vi "Brandon Connection Test.vi"() -> ()   [LabVIEW 2013]
uses:
  <vilib>/Rock Robotics/SystemInterfaces/DIO/FPGA_DIOChannel.ctl
  <vilib>/Rock Robotics/WPI/SPI/WPI_SPIFrameMode.ctl
  <vilib>/Rock Robotics/WPI/SPI/WPI_SPIBits Per Word.ctl
panel:
  out "Binary":bool[](array[boolean])
  out "Received Data":u32
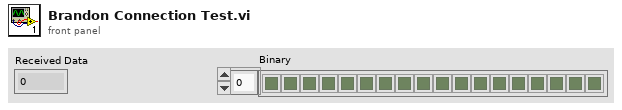
[diagram p1: front panel]
types:
  T1 = typedef "WPI_SPIBits Per Word.ctl" = u8
  T2 = typedef "FPGA_DIOChannel.ctl" = enum8{"DIO 1", "DIO 2", "DIO 3", "DIO 4", "DIO 5", "DIO 6", "DIO 7", "DIO 8", "DIO 9", "DIO 10", "DIO 11", "DIO 12", "DIO 13", "DIO 14", "Invalid"}
  T3 = typedef "WPI_SPIFrameMode.ctl" = enum16{"Chip Select", "Pre-Latch Pulse", "Post-Latch Pulse", "Pre- and Post-Latch Pulse"}
  T4 = typedef "WPI_DigitalOutputDevRef.ctl" = cluster{"Digital Module":T5, "DIO Channel":T2, "DevStatus":errorcluster}
  T5 = typedef "FPGA_TypedefDigitalModule.ctl" = enum16{"Digital Module 1", "Digital Module 2"}
  T6 = typedef "WPI_DigitalInputDevRef.ctl" = cluster{"DevStatus":errorcluster, "DIO Channel":T2, "Digital Module":T5}
  T7 = typedef "WPI_SPIDevRef.ctl" = cluster{"DevStatus":errorcluster}
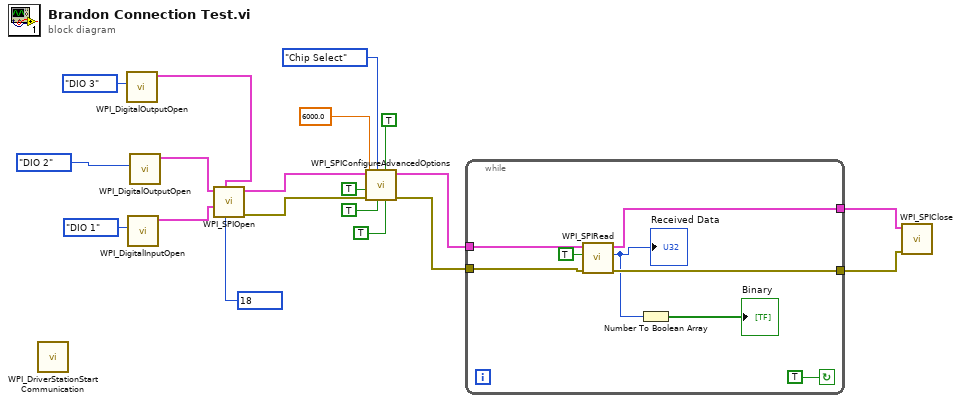
[diagram p0: block diagram]
diagram:
  w1 = T1 18 items=["8-Bit"=8, "16-Bit"=16, "32-Bit"=32] ("Bits Per Word")
  n1 = call <vilib>:"WPI_DriverStationStart Communication.vi"() -> ()  [unwired: 12 in]
  n2 = call <vilib>:"WPI_DigitalOutputOpen.vi"("DIO Channel"=FPGA_DIOChannel."DIO 3") -> ("DigitalOutputDevRef"=w14:T4)  [unwired: 9 in, 1 out]
  n3 = call <vilib>:"WPI_DigitalInputOpen.vi"("DIO Channel"=FPGA_DIOChannel."DIO 1") -> ("DigitalInputDevRef"=w12:T6)  [unwired: 9 in, 1 out]
  n4 = call <vilib>:"WPI_DigitalOutputOpen.vi"("DIO Channel"=FPGA_DIOChannel."DIO 2") -> ("DigitalOutputDevRef"=w15:T4)  [unwired: 9 in, 1 out]
  n5 = call <vilib>:"WPI_SPIOpen.vi"("Bits Per Word"=w1, "Chip Select"=w14, "Master-In Slave-Out"=w12, "Clock"=w15) -> ("error out"=w18:errorcluster, "SPIDevRef"=w19:T7)  [unwired: 6 in]
  n6 = call <vilib>:"WPI_SPIConfigureAdvancedOptions.vi"("Clock Active Low (F)"=TRUE, "Chip Select Active Low (F)"=TRUE, "Clock Phase (Data On Falling) (F)"=TRUE, "Frame Mode (Chip Select)"=WPI_SPIFrameMode."Chip Select", "error in (no error)"=w18, "Most Significant Bit First (F)"=TRUE, "Clock Rate (Hz)"=6000.0, "SPIDevRef"=w19) -> ("error out"=w16:errorcluster, "SPIDevRef"=w17:T7)  [unwired: 2 in]
  n7 = while {
    tunnel: w17 -> [w27]
    tunnel: w16 -> [w26]
    tunnel: [w23] -> w5
    tunnel: [w22] -> w4
    stop <- TRUE continue-if-true
    n8 = call <vilib>:"WPI_SPIRead.vi"("error in (no error)"=w26, "Initiate Transfer (F)"=TRUE, "SPIDevRef"=w27) -> ("error out"=w23:errorcluster, "Received Data"=w21:u32, "SPIDevRef"=w22:T7)  [unwired: 6 in]
    "Received Data" <- w21
    n9 = Number To Boolean Array(number=w21) -> (Boolean array=→"Binary":bool[])
  }
  n10 = call <vilib>:"WPI_SPIClose.vi"("error in (no error)"=w5, "SPIDevRef"=w4) -> ()  [unwired: 9 in, 1 out]
